vi "Teleop_Calc_Actuator.vi"(11 "Teleop Local Data in":T1) -> (3 "Teleop Local Data out":T1)   [LabVIEW 2016]
uses:
  Typedefs/typedef_cluster_Teleop Local Data.ctl
  Typedefs/typedef_enum_Joystick Buttons.ctl
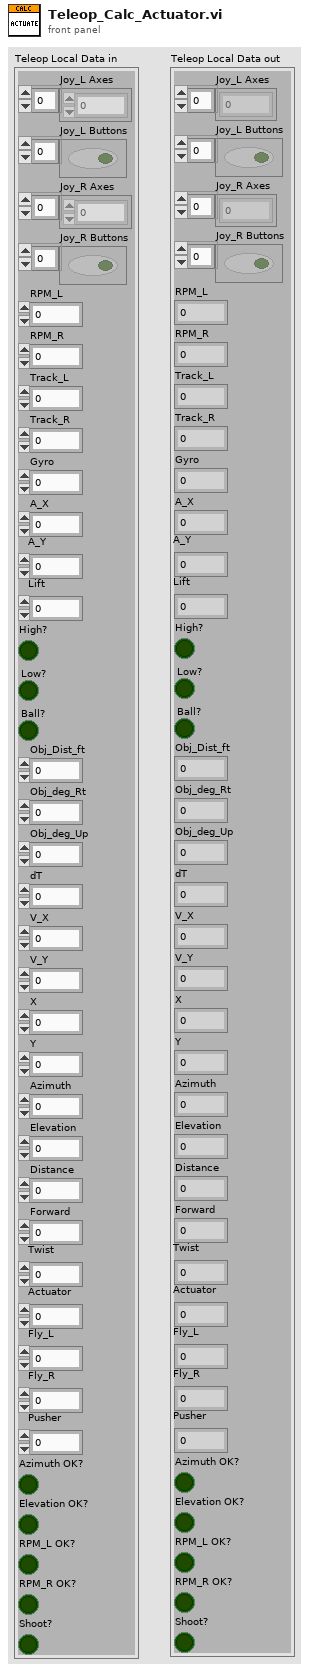
[diagram p1: front panel]
types:
  T1 = typedef "typedef_cluster_Teleop Local Data.ctl" = cluster{"Joy_L Axes":dbl[], "Joy_L Buttons":bool[], "Joy_R Axes":dbl[], "Joy_R Buttons":bool[], "RPM_L":dbl, "RPM_R":dbl, "Track_L":dbl, "Track_R":dbl, "Gyro":dbl, "A_X":dbl, "A_Y":dbl, "Lift":dbl, "High?":bool, "Low?":bool, "Ball?":bool, "Obj_Dist_ft":dbl, "Obj_deg_Rt":dbl, "Obj_deg_Up":dbl, "dT":dbl, "V_X":dbl, "V_Y":dbl, "X":dbl, "Y":dbl, "Azimuth":dbl, "Elevation":dbl, "Distance":dbl, "Forward":dbl, "Twist":dbl, "Actuator":dbl, "Fly_L":dbl, "Fly_R":dbl, "Pusher":dbl, "Azimuth OK?":bool, "Elevation OK?":bool, "RPM_L OK?":bool, "RPM_R OK?":bool, "Shoot?":bool}
  T2 = typedef "typedef_enum_Joystick Buttons.ctl" = enum16{"Trigger", "Thumb", "Top3", "Top4", "Top5", "Top6", "Low7", "Low8", "Low9", "Low10", "Low11", "Low12", "Hat0", "Hat1", "Hat2", "Hat3", "Hat4", "Hat5", "Hat6", "Hat7", "Hat8"}
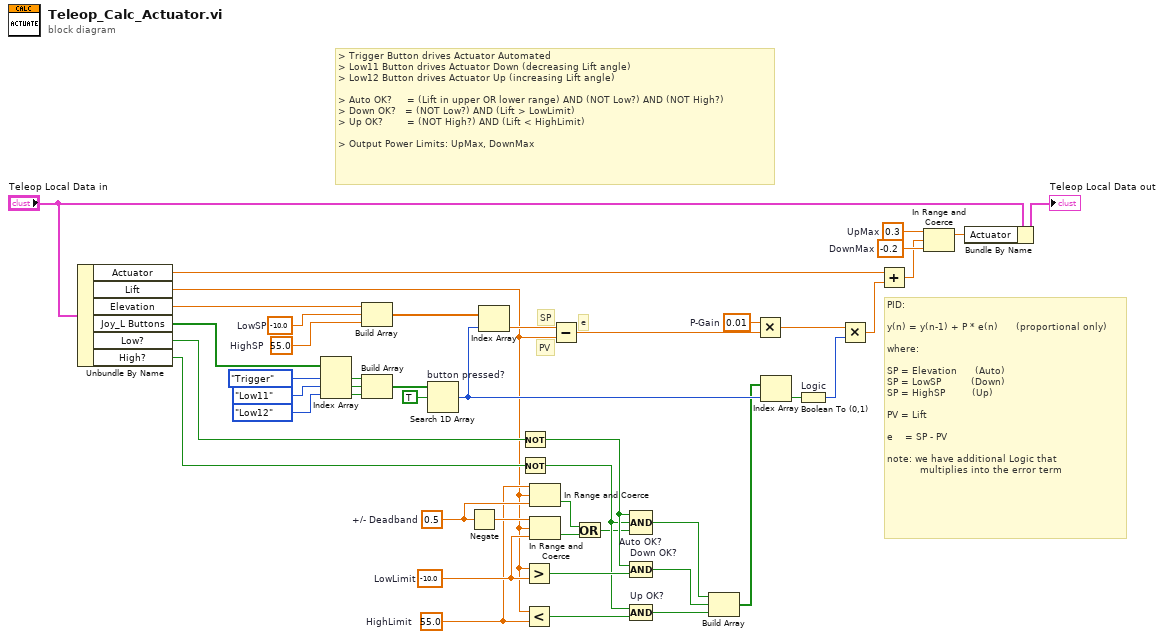
[diagram p0: block diagram]
diagram:
  w28 = 0.01  # P-Gain
  w39 = -10.0  # LowSP
  w38 = 55.0  # HighSP
  w40 = -0.2  # DownMax
  w41 = 0.3  # UpMax
  w15 = 55.0  # HighLimit
  w16 = -10.0  # LowLimit
  w19 = 0.5  # +/- Deadband
  # "PID:\n\ny(n) = y(n-1) + P * e(n)      (proportional only)\n\nwhere:\n\nSP = Elevation      (Auto)\nSP = LowSP          (Down)\nSP = HighSP         (Up)\n\nPV = Lift\n\ne    = SP - PV\n\nnote: we have additional Logic that\n           multiplies into the error term"
  # "e"
  # "PV"
  # "SP"
  # "> Trigger Button drives Actuator Automated\n> Low11 Button drives Actuator Down (decreasing Lift angle)\n> Low12 Button drives Actuator Up (increasing Lift angle)\n\n> Auto OK?     = (Lift in upper OR lower range) AND (NOT Low?) AND (NOT High?)\n> Down OK?   = (NOT Low?) AND (Lift > LowLimit)\n> Up OK?        = (NOT High?) AND (Lift < HighLimit)\n\n> Output Power Limits: UpMax, DownMax"
  n1 = Unbundle By Name("Teleop Local Data in") -> ("Actuator"=w5:dbl, "Lift"=w2:dbl, "Elevation"=w4:dbl, "Joy_L Buttons"=w3:bool[], "Low?"=w44:bool, "High?"=w43:bool)
  n2 = Index Array(array=w3, index #1=typedef_enum_Joystick_Buttons."Trigger" ("Joystick Buttons"), index #2=typedef_enum_Joystick_Buttons."Low11" ("Joystick Buttons"), index #3=typedef_enum_Joystick_Buttons."Low12" ("Joystick Buttons")) -> (element #1=w32:bool, element #2=w36:bool, element #3=w31:bool)
  n3 = Build Array(w4, w39, w38) -> (w26:dbl[])
  n4 = Build Array(w32, w36, w31) -> (w30:bool[])
  n5 = Search 1D Array "button pressed?"(1D array=w30, element=TRUE) -> (index of element=w25:i32)  [unwired: 1 in]
  n6 = Negate(x=w19) -> (-x=w18:dbl)
  n7 = Index Array(array=w26, index=w25) -> (element=w24:dbl)
  n8 = Not(x=w44) -> (.not. x?=w12:bool)
  n9 = Not(x=w43) -> (.not. x?=w11:bool)
  n10 = Greater?(x=w2, y=w16) -> (0:w14:bool)
  n11 = Less?(x=w2, y=w15) -> (x < y?=w13:bool)
  n12 = In Range and Coerce(upper limit=w15, x=w2, lower limit=w19) -> (In Range?=w7:bool)  [unwired: 1 out]
  n13 = In Range and Coerce(upper limit=w18, x=w2, lower limit=w16) -> (In Range?=w17:bool)  [unwired: 1 out]
  n14 = Subtract(x=w24, y=w2) -> (x-y=w29:dbl)
  n15 = Or(x=w7, y=w17) -> (x .or. y?=w6:bool)
  n16 = Compound Arithmetic op=AND "Auto OK?"(w12, w11, w6) -> (w10:bool)
  n17 = Compound Arithmetic op=AND "Down OK?"(w12, w14) -> (w9:bool)
  n18 = Compound Arithmetic op=AND "Up OK?"(w11, w13) -> (w8:bool)
  n19 = Build Array(w10, w9, w8) -> (w1:bool[])
  n20 = Multiply(x=w28, y=w29) -> (x*y=w22:dbl)
  n21 = Index Array(array=w1, index=w25) -> (element=w23:bool)
  n22 = Boolean To (0,1) "Logic"(Boolean=w23) -> (0, 1=w21:i16)
  n23 = Multiply(x=w22, y=w21) -> (x*y=w20:dbl)
  n24 = Add(x=w5, y=w20) -> (x+y=w27:dbl)
  n25 = In Range and Coerce(upper limit=w41, x=w27, lower limit=w40) -> (coerced(x)=w42:dbl)  [unwired: 1 out]
  n26 = Bundle By Name(cluster="Teleop Local Data in", "Actuator"=w42) -> (→"Teleop Local Data out":T1)
